vi "Manuele override.vi"() -> ()   [LabVIEW 2019]
panel:
  out "richtingsaanwijzer":dbl(knob) scale=0.0..10.0
  in  "kruispunt":string
  out "bericht":string
  in  "STOP":bool
  in  "START":bool
  in  "stop 2":bool
  out "address":u32
  out "port":u16
  in  "stop":bool
  in  "vooruit":bool
  in  "achteruit":bool
  in  "links":bool
  in  "rechts":bool
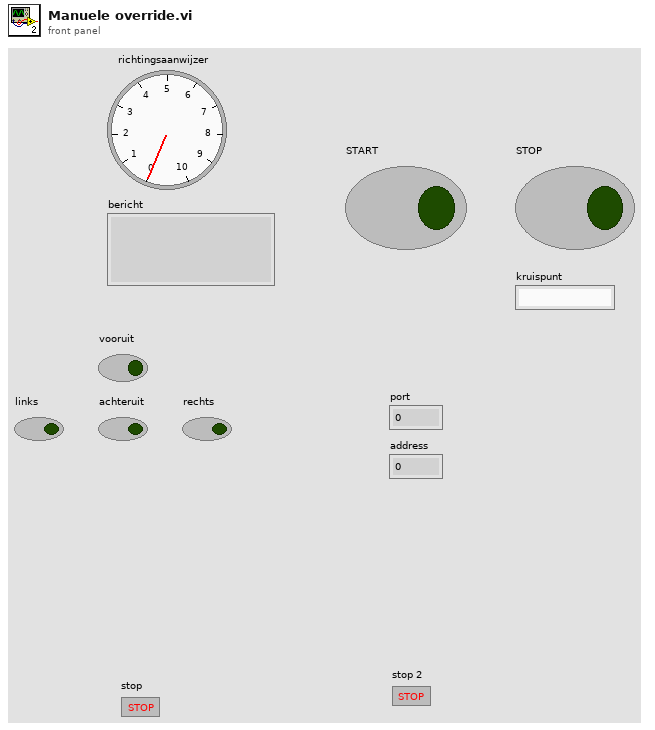
[diagram p1: front panel]
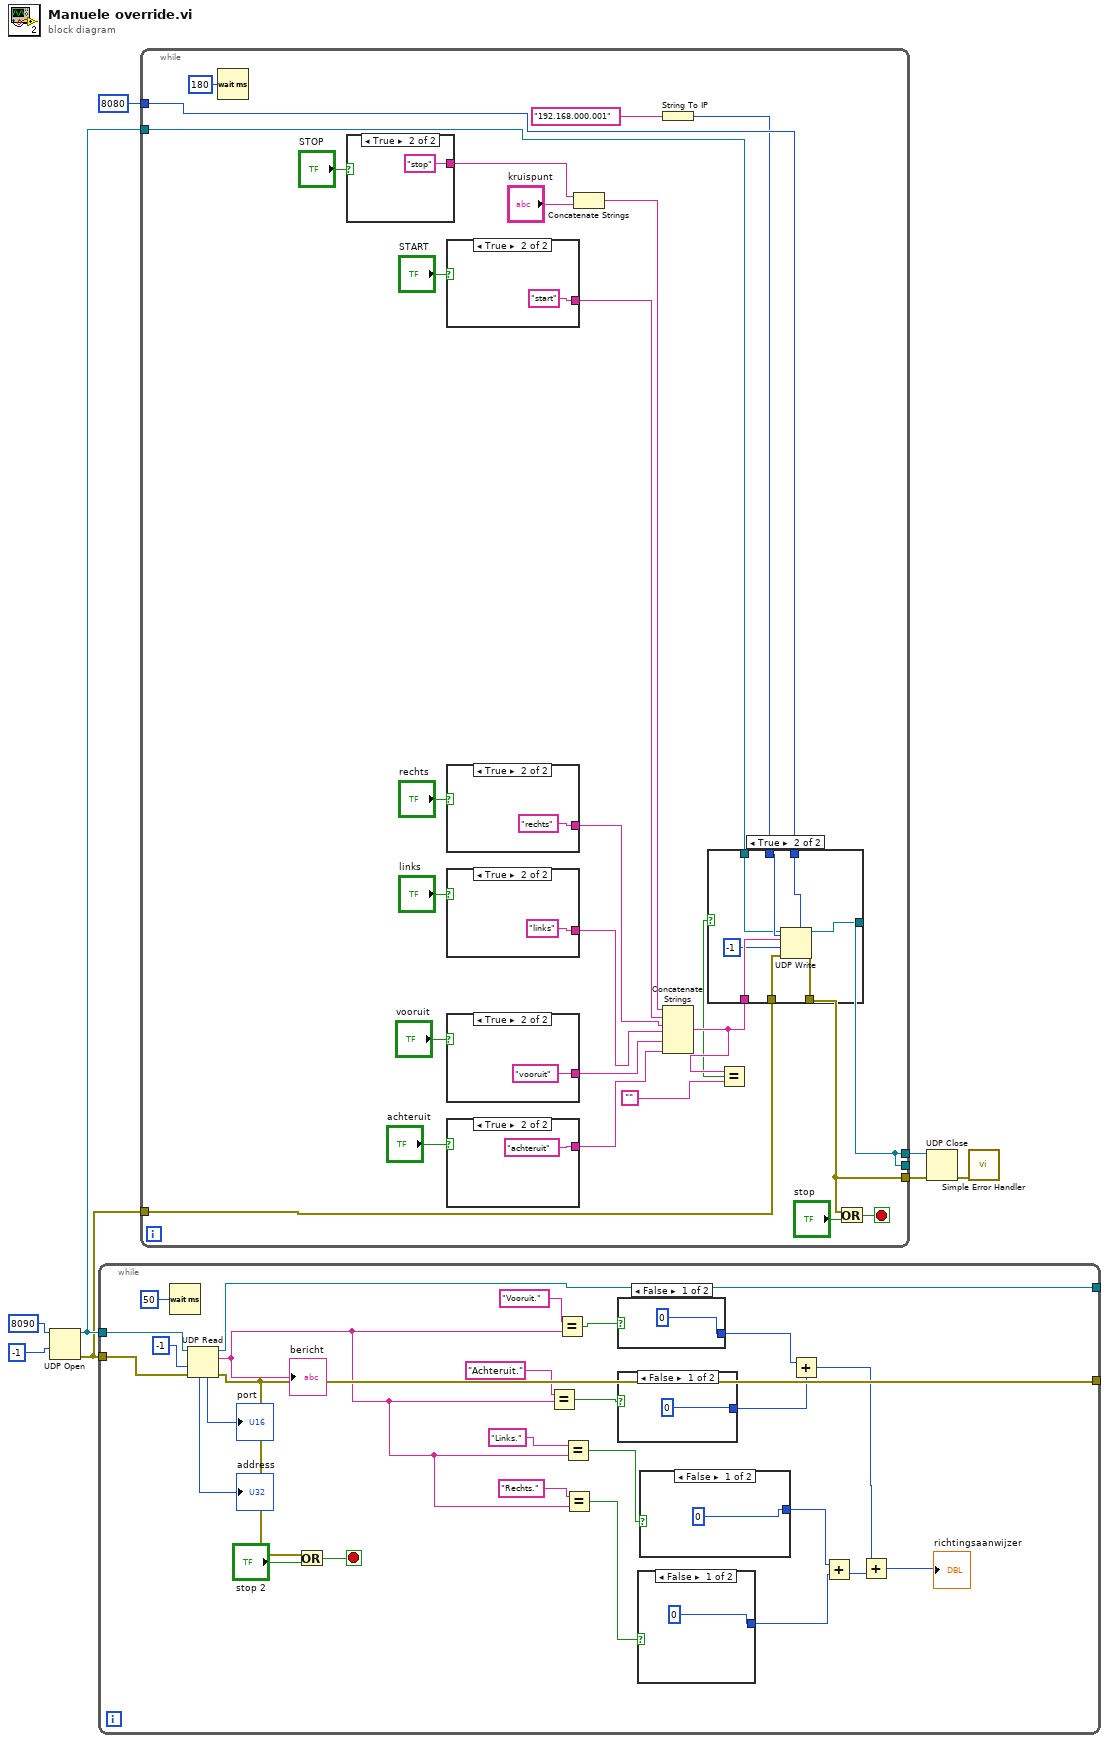
[diagram p0: block diagram]
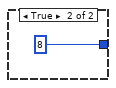
[diagram p2: hidden frame]
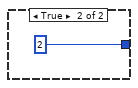
[diagram p3: hidden frame]
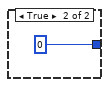
[diagram p4: hidden frame]
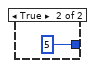
[diagram p5: hidden frame]
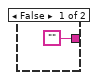
[diagram p7: hidden frame]
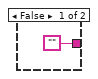
[diagram p8: hidden frame]
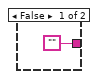
[diagram p9: hidden frame]
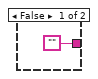
[diagram p10: hidden frame]
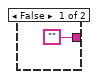
[diagram p11: hidden frame]
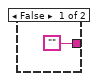
[diagram p12: hidden frame]
diagram:
  n1 = UDP Open(9:-1, 11:8090) -> (port=w4:refnum<k16>, 0:w3:errorcluster)  [unwired: 3 in, 1 out]
  n2 = while {
    tunnel: w4 -> [w34]
    tunnel: w3 -> [w33]
    tunnel: [w30] -> _
    tunnel: [w29] -> _
    stop <- w27 stop-if-true
    n3 = Wait (ms)(milliseconds to wait=u32 50) -> ()  [unwired: 1 out]
    n4 = UDP Read(connection ID=w34, timeout ms (25000)=-1, 8:w33) -> (data out=w19:string, error out=w29:errorcluster, 3:w30:refnum<k16>, 4:→"port":u16, 6:→"address":u32)  [unwired: 1 in]
    "bericht" <- w19
    n5 = Or(x=w29, y="stop 2") -> (x .or. y?=w27:bool)
    n6 = Equal?(x="Achteruit.", y=w19) -> (x = y?=w18:bool)
    n7 = Equal?(x="Vooruit.", y=w19) -> (x = y?=w24:bool)
    n8 = Equal?(x="Links.", y=w19) -> (x = y?=w17:bool)
    n9 = Equal?(x="Rechts.", y=w19) -> (x = y?=w16:bool)
    n10 = case shown="False" w24 {
      tunnel: [0 5] -> w14
      frame False {
      }
      frame True {
      }
    }
    n11 = case shown="False" w18 {
      tunnel: [0 0] -> w15
      frame False {
      }
      frame True {
      }
    }
    n12 = case shown="False" w16 {
      tunnel: [0 8] -> w12
      frame False {
      }
      frame True {
      }
    }
    n13 = case shown="False" w17 {
      tunnel: [0 2] -> w13
      frame False {
      }
      frame True {
      }
    }
    n14 = Add(x=w14, y=w15) -> (x+y=w11:i32)
    n15 = Add(x=w13, y=w12) -> (x+y=w10:i32)
    n16 = Add(x=w11, y=w10) -> (x+y=→"richtingsaanwijzer":i32)
  }
  n17 = while {
    tunnel: w4 -> [w46]
    tunnel: w3 -> [w48]
    tunnel: 8080 -> [w50]
    tunnel: [w44] -> w2
    tunnel: [w45] -> w6
    tunnel: [w44] -> _
    stop <- w68 stop-if-true
    n18 = Wait (ms)(milliseconds to wait=180) -> ()  [unwired: 1 out]
    n19 = case shown="True" "STOP" {
      tunnel: ["" "stop"] -> w57
      frame False {
      }
      frame True {
      }
    }
    n20 = case shown="True" "START" {
      tunnel: ["" "start"] -> w61
      frame False {
      }
      frame True {
      }
    }
    n21 = case shown="True" "rechts" {
      tunnel: ["" "rechts"] -> w55
      frame False {
      }
      frame True {
      }
    }
    n22 = case shown="True" "links" {
      tunnel: ["" "links"] -> w54
      frame False {
      }
      frame True {
      }
    }
    n23 = case shown="True" "vooruit" {
      tunnel: ["" "vooruit"] -> w53
      frame False {
      }
      frame True {
      }
    }
    n24 = case shown="True" "achteruit" {
      tunnel: ["" "achteruit"] -> w52
      frame False {
      }
      frame True {
      }
    }
    n25 = Concatenate Strings(w57, "kruispunt") -> (w58:string)
    n26 = String To IP(1:"192.168.000.001") -> (0:w49:u32)
    n27 = Concatenate Strings(w58, w61, w55, w54, w53, w52) -> (w47:string)
    n28 = Equal?(x=w47, y="") -> (x = y?=w43:bool)
    n29 = case shown="True" w43 {
      tunnel: w50 -> [_ w79]
      tunnel: w49 -> [_ w78]
      tunnel: w48 -> [w71 w77]
      tunnel: w47 -> [_ w76]
      tunnel: w46 -> [w70 w75]
      tunnel: [w71 w74] -> w45
      tunnel: [w70 w73] -> w44
      frame False {
      }
      frame True {
        n30 = UDP Write(address=w78, port or service name=w79, connection ID=w75, data in=w76, 8:w77, 9:-1) -> (error out=w74:errorcluster, 3:w73:refnum<k16>)
      }
    }
    n31 = Or(x=w45, y="stop") -> (x .or. y?=w68:bool)
  }
  n32 = UDP Close(connection ID=w2, 8:w6) -> (error out=w5:errorcluster)  [unwired: 1 out]
  n33 = call <vilib>:"Simple Error Handler.vi"("error in (no error)"=w5) -> ()  [unwired: 4 in, 5 out]
